vi "OA_GetGraph.vi"(4 "Show":bool=TRUE, 5 "Template Name":string="origin", 6 "error in (no error)":errorcluster, 7 "Origin.IOApplication":refnum<k7>) -> (0 "error out":errorcluster, 1 "Origin.GraphLayer":refnum<k7>, 2 "Origin.GraphPage":refnum<k7>, 3 "Origin.IOApplication":refnum<k7>)   [LabVIEW 2010]
doc: "Create an empty graph window\n\nTemplate Name:\n Template file name, .otp extention is not needed.\n if no path is specified, will search Origin folders starting from the \n User Folder, the Group Folder and the Program Folder\nShow:\n Show or Hide the newly added graph window"
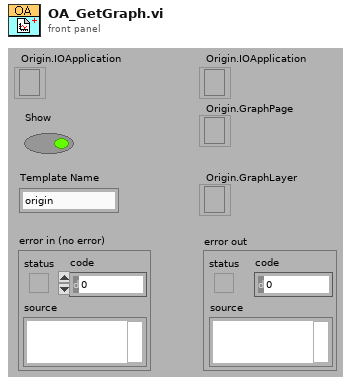
[diagram p1: front panel]
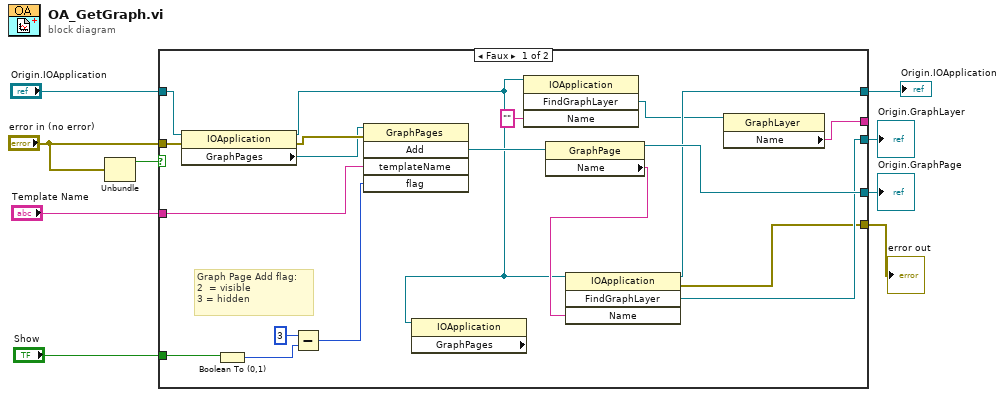
[diagram p0: block diagram]
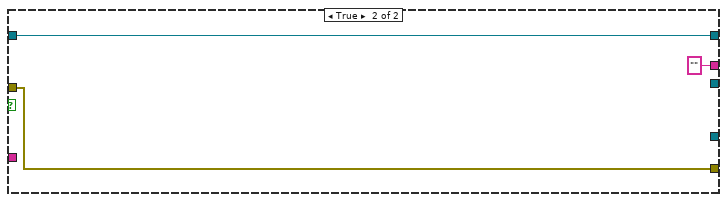
[diagram p2: hidden frame]
diagram:
  n1 = Unbundle("error in (no error)") -> ("status"=w9:bool)  [unwired: 2 out]
  n2 = case shown="Faux" w9 {
    tunnel: "Origin.IOApplication" -> [w27 w31]
    tunnel: [w15 w31] -> w7
    tunnel: "error in (no error)" -> [w28 w30]
    tunnel: "Template Name" -> [w24 _]
    tunnel: "Show" -> [w26 _]
    tunnel: [w16 w30] -> w3
    tunnel: [w20 _] -> w2
    tunnel: [w17 _] -> w1
    tunnel: [w10 "" ("Name")] -> _
    frame False {
      # "Graph Page Add flag: \n2  = visible\n3 = hidden"
      n3 = property class="IOApplication"(reference=w27, error in=w28) -> (reference out=w13:refnum<k7>, error out=w25:errorcluster, "GraphPages"=w14:refnum<k7>)
      n4 = Boolean To (0,1)(Boolean=w26) -> (0, 1=w22:i16)
      n5 = Subtract(x=3, y=w22) -> (x-y=w21:i32)
      n6 = invoke class="GraphPages" method="Add"(reference=w14, error in=w25, "templateName"=w24, "flag"=w21) -> ("Add"=w19:refnum<k7>)  [unwired: 1 in, 4 out]
      n7 = property class="IOApplication" props=["GraphPages"](reference=w13) -> ()  [unwired: 1 in, 3 out]
      n8 = invoke class="IOApplication" method="FindGraphLayer"(reference=w13, "Name"="") -> ("FindGraphLayer"=w11:refnum<k7>)  [unwired: 2 in, 3 out]
      n9 = property class="GraphPage"(reference=w19) -> (reference out=w20:refnum<k7>, "Name"=w18:string)  [unwired: 1 in, 1 out]
      n10 = invoke class="IOApplication" method="FindGraphLayer"(reference=w13, "Name"=w18) -> (reference out=w15:refnum<k7>, error out=w16:errorcluster, "FindGraphLayer"=w17:refnum<k7>)  [unwired: 2 in, 1 out]
      n11 = property class="GraphLayer"(reference=w11) -> ("Name"=w10:string)  [unwired: 1 in, 2 out]
    }
    frame True {
    }
  }
  "Origin.IOApplication" <- w7
  "error out" <- w3
  "Origin.GraphLayer" <- w1
  "Origin.GraphPage" <- w2
